vi "Fit.vi"(8 "error in (no error)":errorcluster caption="entrée d'erreur (pas d'erreur)", 10 "X":cluster{"Key":string[], "Value":i32[]}, 11 "DictVectorizer.lvclass":refnum<class "DictVectorizer.lvclass">) -> (0 "error out":errorcluster caption="sortie d'erreur", 2 "String Data":string, 3 "DictVectorizer.lvclass":refnum<class "DictVectorizer.lvclass">)   [LabVIEW 2020, in "DictVectorizer.lvclass"]
doc: "Learn a list of feature name -> indices mappings.\n\nReturns :\n\n- String : OK"
uses:
  DictVectorizer.lvclass
  DictVectorizer.lvclass/DictVectorizer.ctl
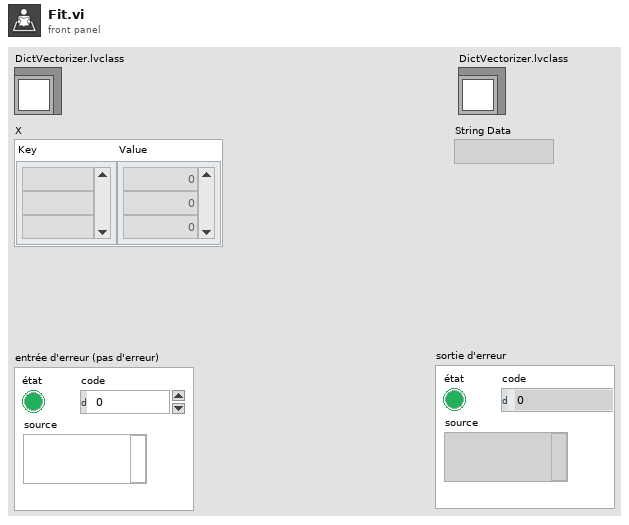
[diagram p1: front panel]
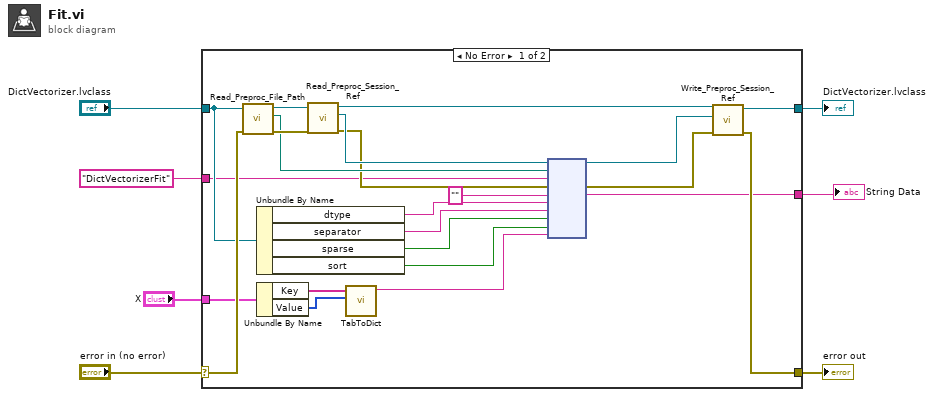
[diagram p0: block diagram]
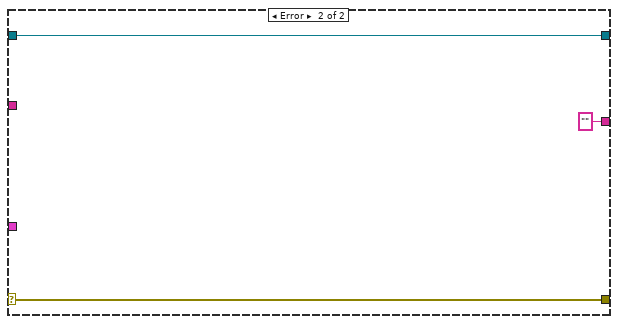
[diagram p2: hidden frame]
diagram:
  n1 = case shown="No Error" "error in (no error)" {
    selector: "error in (no error)" -> [w16 w33]
    tunnel: [w17 w33] -> w6
    tunnel: [w18 w32] -> w4
    tunnel: "DictVectorizer.lvclass" -> [w15 w32]
    tunnel: "DictVectorizerFit" ("Fonction") -> [w14 _]
    tunnel: [w13 ""] -> w2
    tunnel: "X" -> [w10 _]
    frame No Error {
      n2 = call-dynamic "Read_Preproc_File_Path.vi"("error in (no error)"=w16, "Python in"=w15) -> ("error out"=w29:errorcluster, "File_Path"=w28:path, "Python out"=w30:refnum<class "DictVectorizer.lvclass">)  [unwired: 7 in]
      n3 = Unbundle By Name(w15) -> ("dtype"=w21:string, "separator"=w20:string, "sparse"=w19:bool, "sort"=w12:bool)
      n4 = Unbundle By Name(w10) -> ("Key"=w9:string[], "Value"=w11:i32[])
      n5 = call-dynamic "Read_Preproc_Session_Ref.vi"("error in (no error)"=w29, "Python in"=w30) -> ("error out"=w26:errorcluster, "Session_ref"=w27:refnum<k35>, "Python out"=w25:refnum<class "DictVectorizer.lvclass">)  [unwired: 7 in]
      n6 = call "TabToDict.vi"("Int Value"=w11, "String key"=w9) -> ("Dict with int value"=w8:string)  [unwired: 8 in, 1 out]
      n7 = node(w27, w28, w14, w26, "", w21, w20, w19, w12, w8) -> (w23:refnum<k35>, w24:errorcluster, w13:string)  [unwired: 5 in, 2 out]
      n8 = call-dynamic "Write_Preproc_Session_Ref.vi"("error in (no error)"=w24, "Session_ref"=w23, "Python in"=w25) -> ("error out"=w17:errorcluster, "Python out"=w18:refnum<class "DictVectorizer.lvclass">)  [unwired: 7 in]
    }
    frame Error {
    }
  }
  "error out" <- w6
  "DictVectorizer.lvclass" <- w4
  "String Data" <- w2
